vi "Convert version to string.vi"(6 "Ignore Phase":bool, 9 "Version-Numeric":u32) -> (1 "Version-String":string)   [LabVIEW 2016, in "RT Management.lvlib"]
doc: "Converts a numeric version to string."
uses:
  RT Management.lvlib
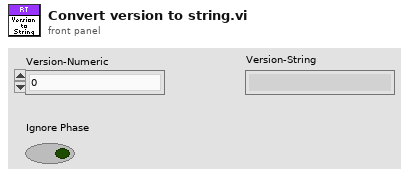
[diagram p1: front panel]
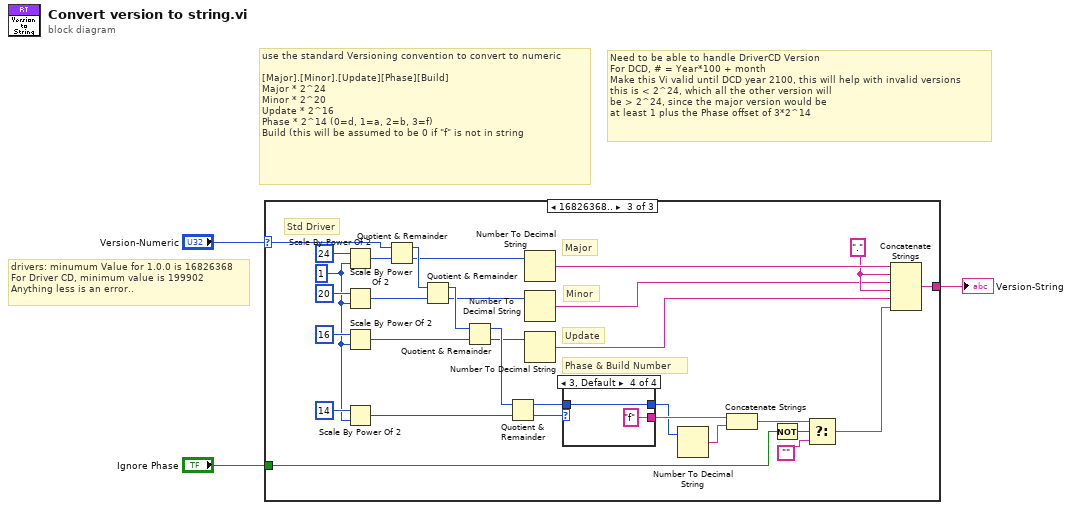
[diagram p0: block diagram]
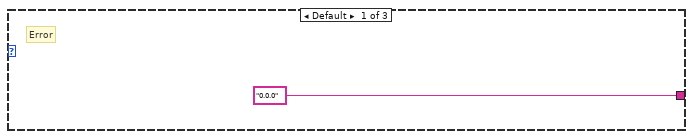
[diagram p2: hidden frame]
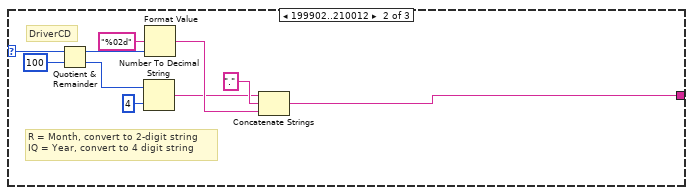
[diagram p3: hidden frame]
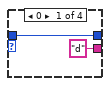
[diagram p4: hidden frame]
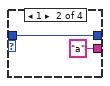
[diagram p5: hidden frame]
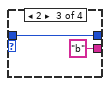
[diagram p6: hidden frame]
diagram:
  # "drivers: minumum Value for 1.0.0 is 16826368\nFor Driver CD, minimum value is 199902\nAnything less is an error.."
  # "Need to be able to handle DriverCD Version\nFor DCD, # = Year*100 + month\nMake this Vi valid until DCD year 2100, this will help with invalid versions\nthis is < 2^24, which all the other version will\nbe > 2^24, since the major version would be\nat least 1 plus the Phase offset of 3*2^14"
  # "use the standard Versioning convention to convert to numeric\n\n[Major].[Minor].[Update][Phase][Build]\nMajor * 2^24\nMinor * 2^20\nUpdate * 2^16\nPhase * 2^14 (0=d, 1=a, 2=b, 3=f)\nBuild (this will be assumed to be 0 if \"f\" is not in string"
  n1 = case shown="16826368.." "Version-Numeric" {
    selector: "Version-Numeric" -> [_ w14 w45]
    tunnel: ["0.0.0" w11 w24] -> w2
    tunnel: "Ignore Phase" -> [_ _ w18]
    frame Default {
      # "Error"
    }
    frame 199902..210012 {
      # "R = Month, convert to 2-digit string\nIQ = Year, convert to 4 digit string"
      # "DriverCD"
      n2 = Quotient & Remainder(x=w14, y=u32 100) -> (x-y*floor(x/y)=w10:u32, floor(x/y)=w7:u32)
      n3 = Number To Decimal String(number=w7, width (-)=i16 4) -> (decimal integer string=w6:string)
      n4 = Format Value(format string="%02d", value (0)=w10) -> (output string=w8:string)  [unwired: 1 out]
      n5 = Concatenate Strings(w6, "." ("string"), w8) -> (w11:string)
    }
    frame 16826368.. {
      w27 = "."
      w39 = u32 1 ("n")
      # "Std Driver"
      # "Phase & Build Number"
      # "Update"
      # "Minor"
      # "Major"
      n6 = Scale By Power Of 2(n=24, x=w39) -> (x*2^n=w43:u32)
      n7 = Scale By Power Of 2(n=20, x=w39) -> (x*2^n=w38:u32)
      n8 = Scale By Power Of 2(n=16, x=w39) -> (x*2^n=w33:u32)
      n9 = Scale By Power Of 2(n=14, x=w39) -> (x*2^n=w34:u32)
      n10 = Quotient & Remainder(x=w45, y=w43) -> (x-y*floor(x/y)=w37:u32, floor(x/y)=w32:u32)
      n11 = Quotient & Remainder(x=w37, y=w38) -> (x-y*floor(x/y)=w36:u32, floor(x/y)=w31:u32)
      n12 = Quotient & Remainder(x=w36, y=w33) -> (x-y*floor(x/y)=w35:u32, floor(x/y)=w30:u32)
      n13 = Quotient & Remainder(x=w35, y=w34) -> (x-y*floor(x/y)=w23:u32, floor(x/y)=w29:u32)
      n14 = Number To Decimal String(number=w32) -> (decimal integer string=w28:string)  [unwired: 1 out]
      n15 = Number To Decimal String(number=w31) -> (decimal integer string=w26:string)  [unwired: 1 out]
      n16 = Number To Decimal String(number=w30) -> (decimal integer string=w25:string)  [unwired: 1 out]
      n17 = case shown="3, Default" w29 {
        tunnel: ["d" "a" "b" "f"] -> w21
        tunnel: w23 -> [w46 w48 w50 w52]
        tunnel: [w46 w48 w50 w52] -> w20
        frame 0 {
        }
        frame 1 {
        }
        frame 2 {
        }
        frame 3, Default {
        }
      }
      n18 = Number To Decimal String(number=w20) -> (decimal integer string=w22:string)  [unwired: 1 out]
      n19 = Concatenate Strings(w21, w22) -> (w19:string)
      n20 = Not(x=w18) -> (.not. x?=w17:bool)
      n21 = Select(t=w19, s=w17, f="") -> (s? t:f=w15:string)
      n22 = Concatenate Strings(w28, w27, w26, w27, w25, w15) -> (w24:string)
    }
  }
  "Version-String" <- w2
